vi "F Dwf Analog Out Node Play Status.vi"(0 "hdwf":i32, 1 "cdDataLost":i32, 5 "idxChannel":i32, 7 "node":i32, 9 "cdDataFree":i32, 11 "error in (no error)":errorcluster, 12 "cdDataCorrupted":i32) -> (3 "cdDataLost out":i32, 4 "function return":i32, 10 "cdDataFree out":i32, 14 "cdDataCorrupted out":i32, 15 "error out":errorcluster)   [LabVIEW 2021, in "Olasdwf.lvlib"]
doc: "DWFAPI int FDwfAnalogOutNodePlayStatus(HDWF hdwf, int idxChannel, AnalogOutNode node, int *cdDataFree, int *cdDataLost, int *cdDataCorrupted);"
uses:
  Olasdwf.lvlib
  Windows/System32/dwf.dll
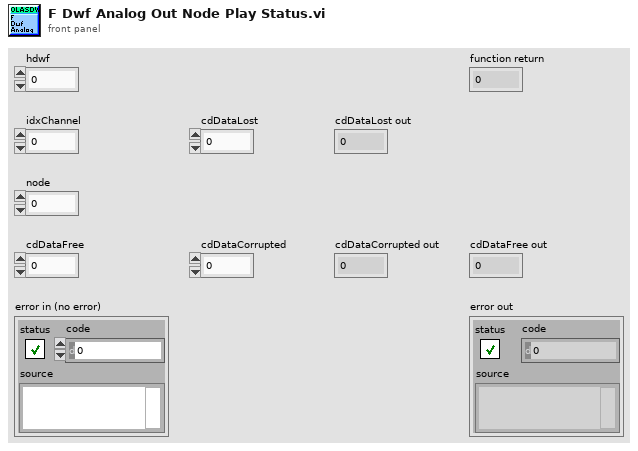
[diagram p1: front panel]
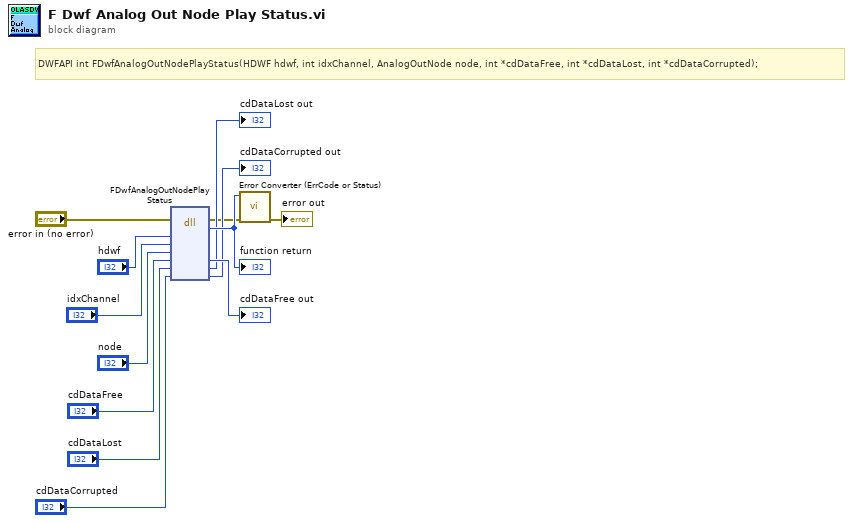
[diagram p0: block diagram]
diagram:
  # "DWFAPI int FDwfAnalogOutNodePlayStatus(HDWF hdwf, int idxChannel, AnalogOutNode node, int *cdDataFree, int *cdDataLost, int *cdDataCorrupted);"
  n1 = dll-call lib="/Windows/System32/dwf.*" fn="FDwfAnalogOutNodePlayStatus"(error in="error in (no error)", "hdwf"="hdwf", "idxChannel"="idxChannel", "node"="node", "cdDataFree"="cdDataFree", "cdDataLost"="cdDataLost", "cdDataCorrupted"="cdDataCorrupted") -> (error out=w2:errorcluster, w13:i32, "cdDataFree"=→"cdDataFree out":i32, "cdDataLost"=→"cdDataLost out":i32, "cdDataCorrupted"=→"cdDataCorrupted out":i32)  [unwired: 5 in, 1 out]
  "function return" <- w13
  n2 = call "Error Converter (ErrCode or Status).vi"("error in (no error)"=w2, "error code"=w13) -> ("error out"=→"error out":errorcluster)  [unwired: 9 in]
